vi "absCalcPlot_III.vi"(6 "Cell Calibration, mV/mW":dbl=600000.0, 8 "Error In":errorcluster, 9 "PD Values":cluster{dbl, dbl, dbl}, 10 "bkg values":cluster{dbl, dbl, dbl}, 11 "Mic Values":cluster{dbl, dbl, dbl}) -> (0 "Error Out":errorcluster, 1 "aae":dbl, 2 "Time Series":cluster{dbl, dbl, dbl}, 3 "Spectrum":cluster{dbl[], "Best Power Fit":dbl[]}[](graph))   [LabVIEW 2011]
uses:
  <vilib>/Analysis/NI_AALPro.lvlib
panel:
  out "output cluster":cluster{i32[], "Best Power Fit":dbl[]}
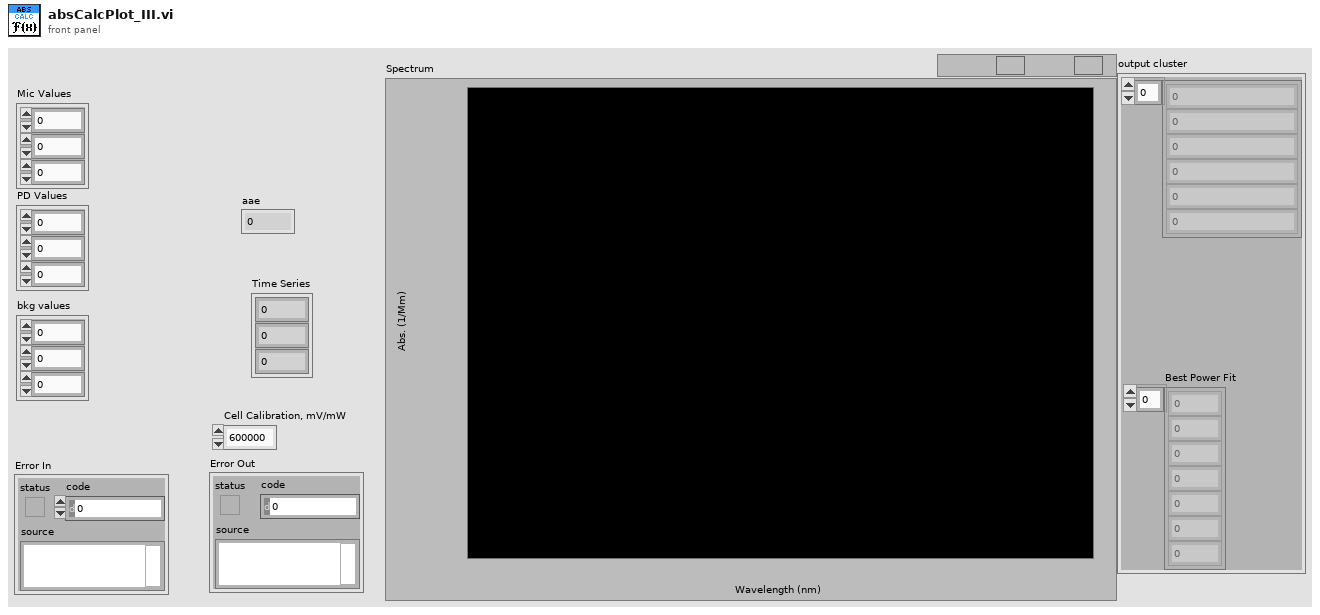
[diagram p1: front panel]
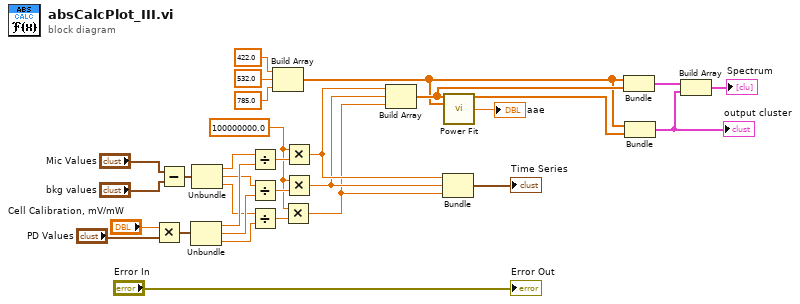
[diagram p0: block diagram]
diagram:
  w9 = 100000000.0 ("element")
  n1 = Multiply(x="Cell Calibration, mV/mW", y="PD Values") -> (x*y=w25:cluster{dbl, dbl, dbl})
  n2 = Subtract(x="Mic Values", y="bkg values") -> (x-y=w17:cluster{dbl, dbl, dbl})
  n3 = Unbundle(w25) -> (w26:dbl, w27:dbl, w28:dbl)
  n4 = Unbundle(w17) -> (w20:dbl, w21:dbl, w22:dbl)
  n5 = Divide(x=w20, y=w26) -> (x/y=w12:dbl)
  n6 = Divide(x=w21, y=w27) -> (x/y=w11:dbl)
  n7 = Divide(x=w22, y=w28) -> (x/y=w10:dbl)
  n8 = Build Array(422.0 ("element"), 532.0 ("element"), 785.0 ("element")) -> (w6:dbl[])
  n9 = Multiply(x=w9, y=w10) -> (x*y=w2:dbl)
  n10 = Multiply(x=w9, y=w12) -> (x*y=w4:dbl)
  n11 = Multiply(x=w9, y=w11) -> (x*y=w3:dbl)
  n12 = Build Array(w4, w3, w2) -> (w7:dbl[])
  n13 = Bundle(w4, w3, w2) -> (→"Time Series":cluster{dbl, dbl, dbl})  [unwired: 1 in]
  n14 = call <vilib>:"Power Fit.vi"("Y"=w7, "X"=w6) -> ("Best Power Fit"=w15:dbl[], "power"=→"aae":dbl)  [unwired: 8 in, 4 out]
  n15 = Bundle(w6, w7) -> (w5:cluster{dbl[], dbl[]})  [unwired: 1 in]
  n16 = Bundle(w6, "Best Power Fit"=w15) -> (w14:cluster{dbl[], "Best Power Fit":dbl[]})  [unwired: 1 in]
  "output cluster" <- w14
  n17 = Build Array(w5, w14) -> (→"Spectrum":cluster{dbl[], "Best Power Fit":dbl[]}[])
  "Error Out" <- "Error In"
